vi "acqTime.vi"(8 "error in":errorcluster) -> (0 "error out":errorcluster, 2 "Loop time":u16)   [LabVIEW 2020]
uses:
  <vilib>/ptbypt/NI_PtbyPt.lvlib
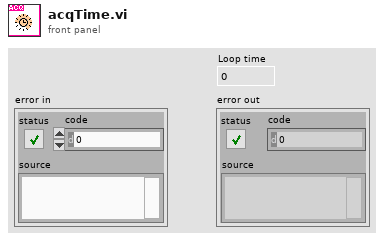
[diagram p1: front panel]
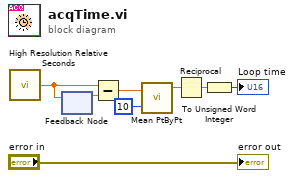
[diagram p0: block diagram]
diagram:
  n1 = call <vilib>:"High Resolution Relative Seconds.vi"() -> ("relative seconds"=w7:dbl)
  n2 = feedback #1() -> (w8:dbl)  [unwired: 1 in]
  n3 = feedback-in #1(w7) -> ()
  n4 = Subtract(x=w7, y=w8) -> (x-y=w3:dbl)
  n5 = call <vilib>:"Mean PtByPt.vi"("x"=w3, "sample length"=10) -> ("mean"=w6:dbl)  [unwired: 2 in, 1 out]
  n6 = Reciprocal(x=w6) -> (1/x=w5:dbl)
  n7 = To Unsigned Word Integer(number=w5) -> (unsigned 16bit integer=→"Loop time":u16)
  "error out" <- "error in"
